vi "RSD Command Read.vi"(0 "VISA resource name":refnum<visa-resource-name>, 1 "Checksum used":bool=TRUE, 5 "Responce":string, 11 "error in (no error)":errorcluster) -> (3 "STX":string, 4 "VISA resource name out":refnum<visa-resource-name>, 6 "OK":string, 8 "Value (string)":string, 10 "Value (decimal)":u32, 12 "Address":string, 13 "Command":string, 14 "Checksum":string, 15 "error out":errorcluster)   [LabVIEW 2017, in "Samwontech TEMP2xxx.lvlib"]
uses:
  <instrlib>/Samwontech TEMP2xxx/Samwontech TEMP2xxx.lvlib
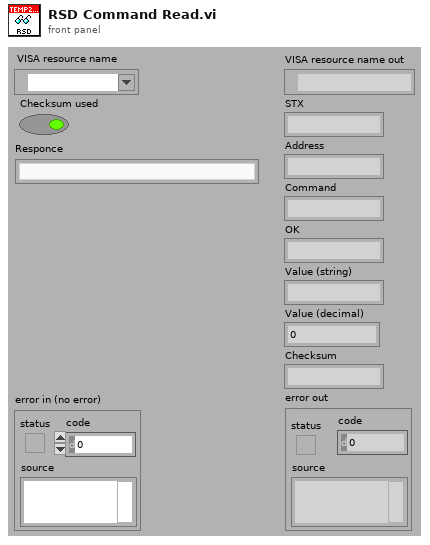
[diagram p1: front panel]
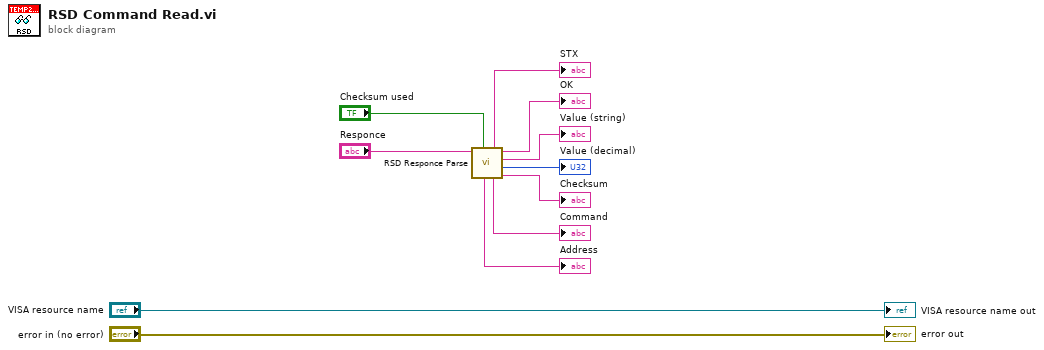
[diagram p0: block diagram]
diagram:
  n1 = call <instrlib>:"RSD Responce Parse.vi"("Checksum used"="Checksum used", "Responce"="Responce") -> ("Checksum"=→"Checksum":string, "Value (decimal)"=→"Value (decimal)":u32, "Value (string)"=→"Value (string)":string, "OK"=→"OK":string, "Command"=→"Command":string, "STX"=→"STX":string, "Address"=→"Address":string)  [unwired: 3 in]
  "error out" <- "error in (no error)"
  "VISA resource name out" <- "VISA resource name"
